vi "Grpahing2.vi"() -> ()   [LabVIEW 2021]
panel:
  out "Signal-Vg":cluster{dbl, dbl, dbl}[](graph)
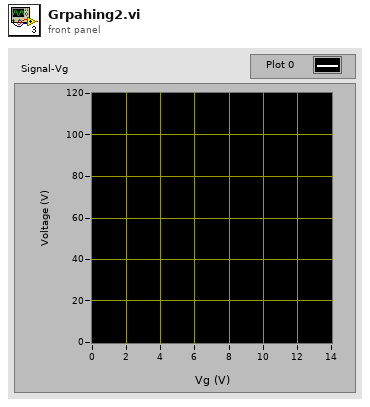
[diagram p1: front panel]
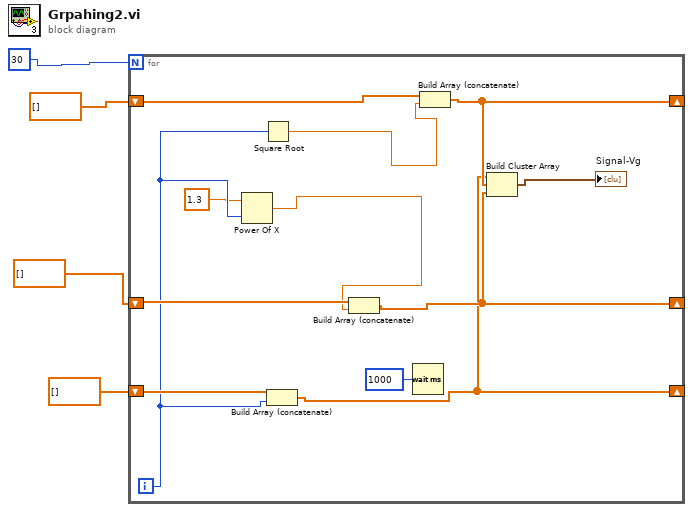
[diagram p0: block diagram]
diagram:
  n1 = for {
    N: 30 -> [_]
    shift-right: [w12] -> _
    shift-left: dbl[] [] -> [w15]
    shift-right: [w11] -> _
    shift-left: dbl[] [] -> [w14]
    shift-right: [w8] -> _
    shift-left: dbl[] [] -> [w9]
    i -> [w6]
    n2 = Power Of X(1:w6, 2:1.3 ("y")) -> (0:w7:dbl)
    n3 = Square Root(x=w6) -> (sqrt(x)=w13:dbl)
    n4 = Build Array (concatenate)(w9, w6) -> (w8:dbl[])
    n5 = Build Array (concatenate)(w14, w7) -> (w11:dbl[])
    n6 = Wait (ms)(milliseconds to wait=u32 1000) -> ()  [unwired: 1 out]
    n7 = Build Array (concatenate)(w15, w13) -> (w12:dbl[])
    n8 = Build Cluster Array(w8, w12, w11) -> (→"Signal-Vg":cluster{dbl, dbl, dbl}[])
  }
